vi "test_amplitude_limit.vi"() -> ()   [LabVIEW 2018]
panel:
  in  "enabled":bool
  out "x/y I":dbl
  in  "Limit":fxp<+/-,32,14>=512.0 format="%#_23g"
  out "x/y Q":dbl
  out "A^2":dbl
  out "sqrt(x)":dbl
  out "Waveform Graph":i16[](graph)
  out "Array":bool[](array[boolean])
  in  "Data in":fxp<+/-,32,14>[](array[numeric])=[0.0, 0.0]
  out "Data out":fxp<+/-,32,14>[](array[numeric])
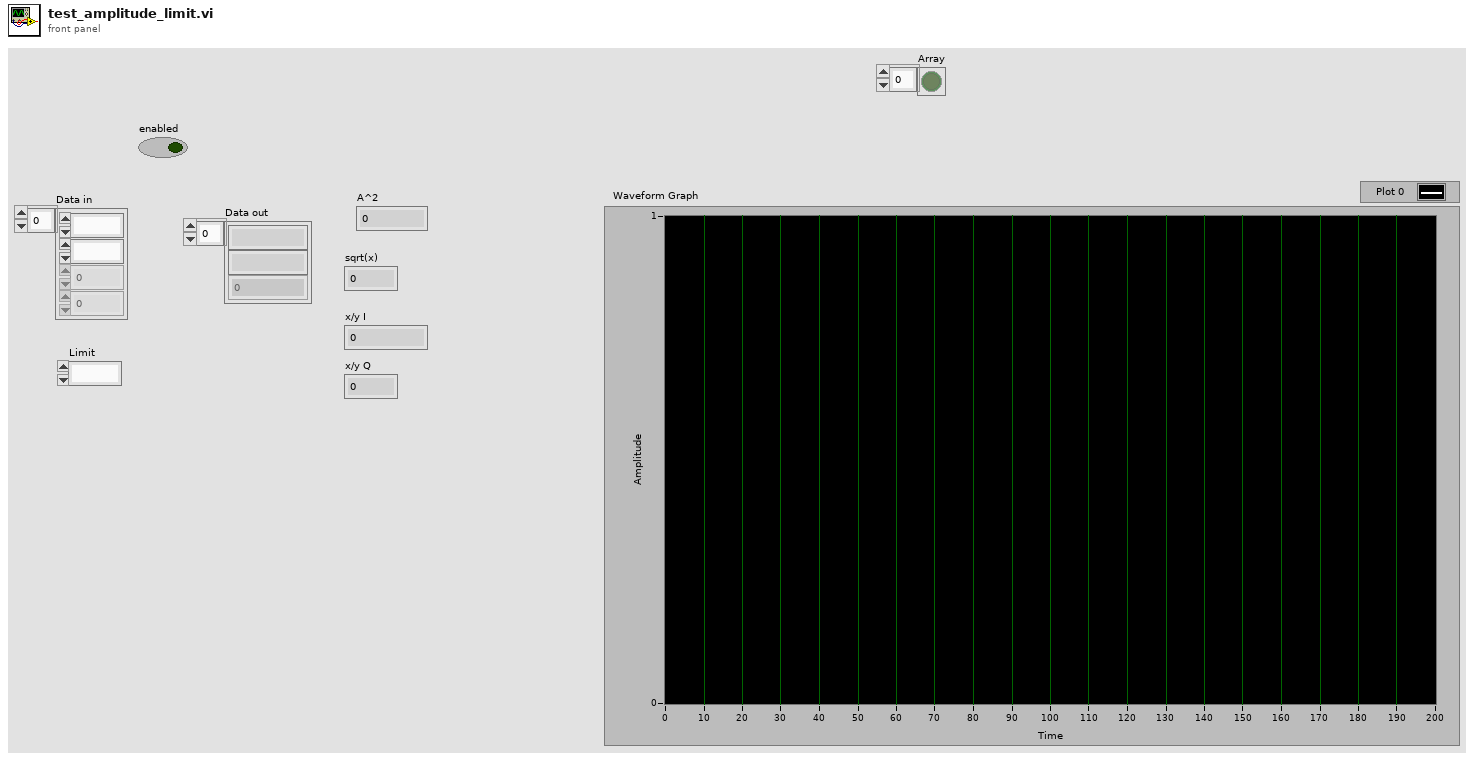
[diagram p1: front panel]
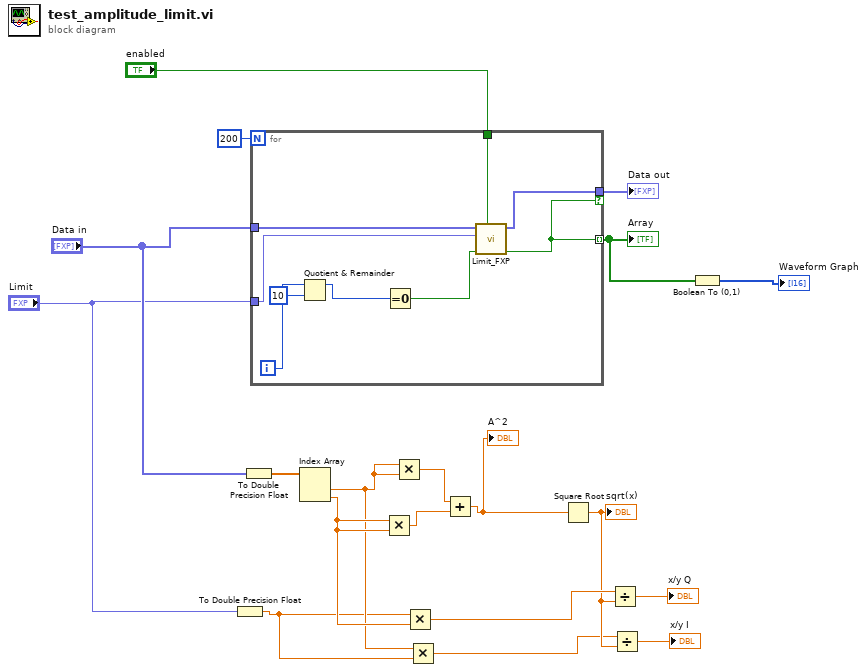
[diagram p0: block diagram]
diagram:
  n1 = To Double Precision Float(number="Limit") -> (double precision float=w3:dbl)
  n2 = To Double Precision Float(number="Data in") -> (double precision float=w14:dbl[])
  n3 = for {
    N: 200 -> [_]
    tunnel: [w21] -> w17 mode=indexing
    tunnel: "Data in" -> [w24]
    tunnel: [w23] -> w18 if=w21
    tunnel: "Limit" -> [w22]
    tunnel: "enabled" -> [w20]
    i -> [w28]
    n4 = Quotient & Remainder(x=w28, y=10) -> (x-y*floor(x/y)=w26:i32)  [unwired: 1 out]
    n5 = Equal To 0?(x=w26) -> (x = 0?=w25:bool)
    n6 = call "Limit_FXP.vi"("enabled"=w20, "input valid"=w25, "Limit"=w22, "Data in"=w24) -> ("output valid"=w21:bool, "Data out"=w23:fxp<+/-,32,14>[])  [unwired: 6 in]
  }
  "Data out" <- w18
  "Array" <- w17
  n7 = Index Array(array=w14) -> (element #1=w4:dbl, element #2=w9:dbl)  [unwired: 2 in]
  n8 = Multiply(x=w9, y=w9) -> (x*y=w12:dbl)
  n9 = Multiply(x=w4, y=w4) -> (x*y=w13:dbl)
  n10 = Multiply(x=w3, y=w9) -> (x*y=w8:dbl)
  n11 = Multiply(x=w4, y=w3) -> (x*y=w2:dbl)
  n12 = Add(x=w13, y=w12) -> (x+y=w11:dbl)
  "A^2" <- w11
  n13 = Square Root(x=w11) -> (sqrt(x)=w5:dbl)
  "sqrt(x)" <- w5
  n14 = Divide(x=w8, y=w5) -> (x/y=→"x/y Q":dbl)
  n15 = Divide(x=w2, y=w5) -> (x/y=→"x/y I":dbl)
  n16 = Boolean To (0,1)(Boolean=w17) -> (0, 1=→"Waveform Graph":i16[])
